vi "OpenDBL.vi"(2 "Action":u16(ring) items=["Get Image", "Load and Read File"]) -> (4 "Image":sgl[](array[numeric]), 8 "Physical Length (Z, Y, X, t)":sgl[](array[numeric]), 13 "File Notes":string, 15 "Dimensions (Z, Y, X, t)":i32[](array[numeric]))   [LabVIEW 2014]
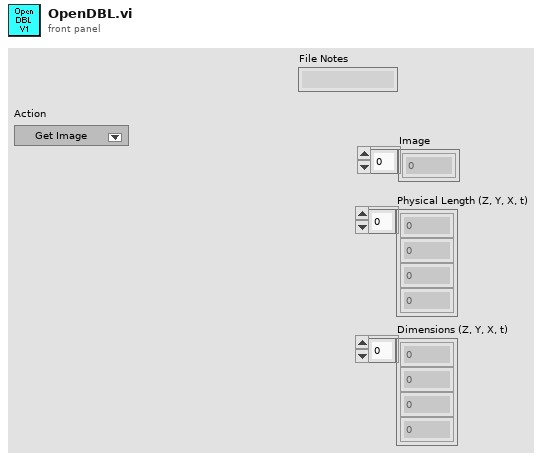
[diagram p1: front panel]
types:
  T1 = enum16{"big-endian, network order", "native, host order", "little-endian"}
  T2 = enum16{"open", "replace", "create", "open or create", "replace or create", "replace or create with confirmation"}
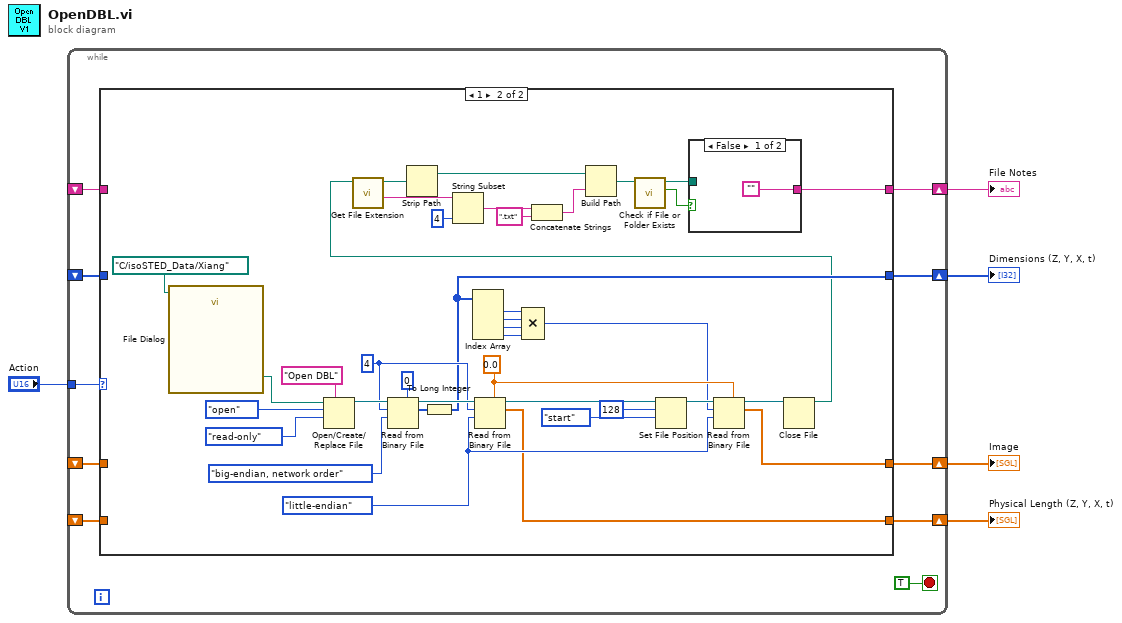
[diagram p0: block diagram]
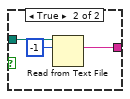
[diagram p3: hidden frame]
diagram:
  n1 = while {
    shift-right: [w13] -> w2
    shift-left: _ -> [w10]
    shift-right: [w11] -> w3
    shift-left: _ -> [w9]
    shift-right: [w12] -> w4
    shift-left: _ -> [w8]
    tunnel: "Action" -> [w14]
    shift-right: [w7] -> w1
    shift-left: _ -> [w6]
    stop <- TRUE stop-if-true
    n2 = case shown="1" w14 {
      tunnel: [w17 w41] -> w12
      tunnel: [w19 w35] -> w13
      tunnel: [w18 w39] -> w11
      tunnel: w10 -> [w19 _]
      tunnel: w9 -> [w18 _]
      tunnel: w8 -> [w17 _]
      tunnel: [w16 w22] -> w7
      tunnel: w6 -> [w16 _]
      frame 0, Default {
      }
      frame 1 {
        w47 = sgl 0.0
        w45 = T1."little-endian" ("byte order (0:big-endian, network order)")
        w48 = 4 ("count (1)")
        n3 = call "File Dialog"("start path"=path "C:/isoSTED_Data/Xiang") -> ("selected path"=w21:path)  [unwired: 11 in, 3 out]
        n4 = Open/Create/Replace File(file path (use dialog)=w21, prompt="Open DBL", operation (0:open)=T2."open", access (0:read/write)=enum16{"read/write", "read-only", "write-only"}."read-only") -> (refnum out=w54:refnum<file>)  [unwired: 2 in, 2 out]
        n5 = Read from Binary File(5:u16 0, 9:T1."big-endian, network order" ("byte order (0:big-endian, network order)"), 10:w48, 11:w54) -> (2:w40:u16[], 3:w51:refnum<file>)  [unwired: 2 in, 2 out]
        n6 = To Long Integer(number=w40) -> (32bit integer=w35:i32[])
        n7 = Index Array(array=w35) -> (element #1=w36:i32, element #2=w37:i32, element #3=w43:i32, element #4=w42:i32)  [unwired: 4 in]
        n8 = Read from Binary File(5:w47, 9:w45, 10:w48, 11:w51) -> (2:w41:sgl[], 3:w50:refnum<file>)  [unwired: 2 in, 2 out]
        n9 = Compound Arithmetic op=MULTIPLY(w36, w37, w43, w42) -> (w34:i32)
        n10 = Set File Position(offset (in bytes) (0)=i64 128, refnum=w50, from (0:start)=enum16{"start", "end", "current"}."start") -> (refnum out=w38:refnum<file>)  [unwired: 1 in, 1 out]
        n11 = Read from Binary File(5:w47, 9:w45, 10:w34, 11:w38) -> (2:w39:sgl[], 3:w44:refnum<file>)  [unwired: 2 in, 2 out]
        n12 = Close File(refnum=w44) -> (path=w23:path)  [unwired: 1 in, 1 out]
        n13 = call <vilib>:"Get File Extension.vi"("file"=w23) -> ("filename without extension"=w25:string, "dup file"=w24:path)  [unwired: 7 in, 2 out]
        n14 = Strip Path(path=w24) -> (stripped path=w28:path)  [unwired: 1 out]
        n15 = String Subset(string=w25, length (rest)=4 ("length (rest)")) -> (substring=w26:string)  [unwired: 1 in]
        n16 = Concatenate Strings(w26, ".txt" ("string")) -> (w29:string)
        n17 = Build Path(base path=w28, name or relative path=w29) -> (appended path=w31:path)
        n18 = call <vilib>:"Check if File or Folder Exists.vi"("path"=w31) -> ("file or folder exists?"=w33:bool, "dup path"=w32:path)  [unwired: 8 in, 1 out]
        n19 = case shown="False" w33 {
          tunnel: w32 -> [_ w60]
          tunnel: ["" w59] -> w22
          frame False {
          }
          frame True {
            n20 = Read from Text File(file (use dialog)=w60, count=-1) -> (text=w59:string)  [unwired: 2 in, 3 out]
          }
        }
      }
    }
  }
  "Dimensions (Z, Y, X, t)" <- w2
  "Physical Length (Z, Y, X, t)" <- w4
  "Image" <- w3
  "File Notes" <- w1
